vi "U8_3_byte_Array_to_voltage_current_Rev01.vi"(10 "Array In":u8[](array[numeric]), 11 "Nmbr_of_datasamples":dbl=128.0) -> (0 "Current":dbl[](graph), 1 "mV":dbl, 2 "Voltage":dbl[](graph), 3 "Loop count":dbl, 4 "COM":dbl[](graph), 6 "HEXVAL":string)   [LabVIEW 2012]
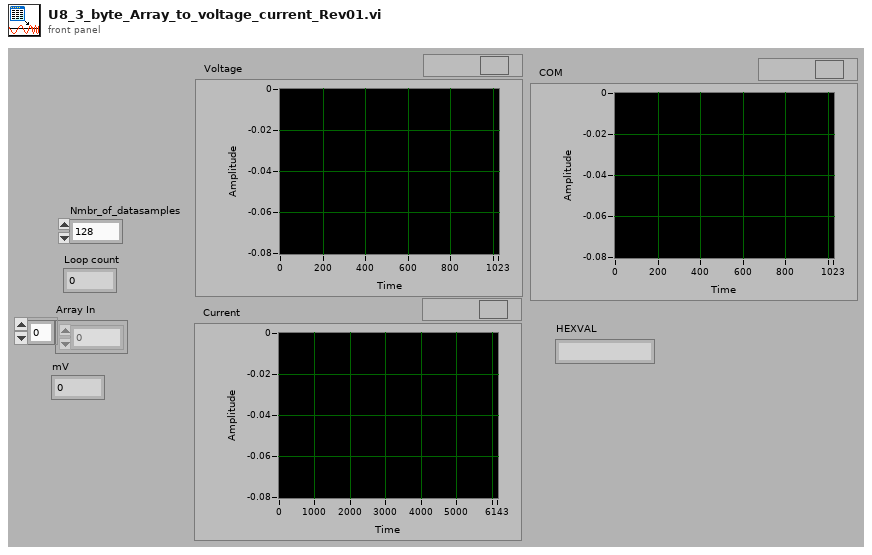
[diagram p1: front panel]
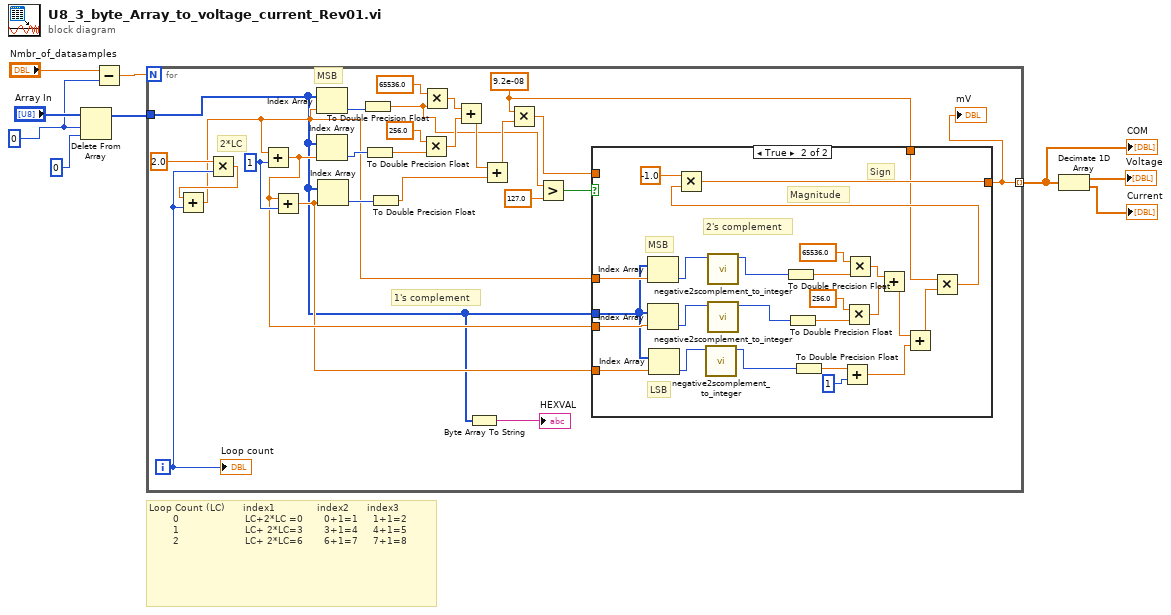
[diagram p0: block diagram]
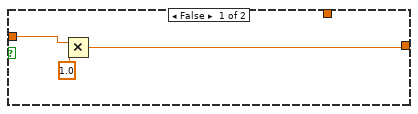
[diagram p2: hidden frame]
diagram:
  w5 = 0
  # "Loop Count (LC)      index1              index2      index3      \n        0                      LC+2*LC =0       0+1=1     1+1=2\n        1                      LC+ 2*LC=3       3+1=4     4+1=5\n        2                      LC+ 2*LC=6       6+1=7     7+1=8"
  n1 = Delete From Array(array="Array In", length=w5, index=0) -> (array with subset deleted=w4:u8[])  [unwired: 1 out]
  n2 = Subtract(x="Nmbr_of_datasamples", y=w5) -> (x-y=w7:dbl)
  n3 = for {
    N: w7 -> [_]
    tunnel: w4 -> [w10]
    tunnel: [w12] -> w1 mode=indexing
    i -> [w17]
    w16 = 9.2e-08
    w27 = 1
    # "1's complement"
    # "MSB"
    # "2*LC"
    n4 = Multiply(x=2.0, y=w17) -> (x*y=w25:dbl)
    n5 = Add(x=w25, y=w17) -> (x+y=w15:dbl)
    n6 = Add(x=w15, y=w27) -> (x+y=w14:dbl)
    n7 = Add(x=w14, y=w27) -> (x+y=w13:dbl)
    n8 = Index Array(array=w10, index=w15) -> (element=w20:u8)
    n9 = Index Array(array=w10, index=w14) -> (element=w19:u8)
    n10 = Index Array(array=w10, index=w13) -> (element=w18:u8)
    n11 = To Double Precision Float(number=w20) -> (double precision float=w21:dbl)
    n12 = To Double Precision Float(number=w19) -> (double precision float=w33:dbl)
    n13 = To Double Precision Float(number=w18) -> (double precision float=w29:dbl)
    n14 = Multiply(x=256.0, y=w33) -> (x*y=w31:dbl)
    n15 = Multiply(x=65536.0, y=w21) -> (x*y=w35:dbl)
    n16 = Add(x=w35, y=w31) -> (x+y=w30:dbl)
    n17 = Byte Array To String(unsigned byte array=w10) -> (string=→"HEXVAL":string)
    n18 = Add(x=w30, y=w29) -> (x+y=w28:dbl)
    n19 = Multiply(x=w16, y=w28) -> (x*y=w24:dbl)
    n20 = Greater?(x=w21, y=127.0) -> (0:w23:bool)
    n21 = case shown="True" w23 {
      tunnel: [w38 w63] -> w12
      tunnel: w24 -> [w37 _]
      tunnel: w10 -> [_ w48]
      tunnel: w15 -> [_ w53]
      tunnel: w14 -> [_ w52]
      tunnel: w13 -> [_ w51]
      tunnel: w16 -> [_ w49]
      frame False {
        n22 = Multiply(x=w37, y=1.0) -> (x*y=w38:dbl)
      }
      frame True {
        # "LSB"
        # "Magnitude"
        # "Sign"
        # "2's complement"
        # "MSB"
        n23 = Index Array(array=w48, index=w53) -> (element=w47:u8)
        n24 = Index Array(array=w48, index=w52) -> (element=w45:u8)
        n25 = Index Array(array=w48, index=w51) -> (element=w43:u8)
        n26 = call "negative2scomplement_to_integer.vi"("BYTE"=w43) -> ("Result"=w42:u8)  [unwired: 10 in]
        n27 = call "negative2scomplement_to_integer.vi"("BYTE"=w47) -> ("Result"=w46:u8)  [unwired: 10 in]
        n28 = call "negative2scomplement_to_integer.vi"("BYTE"=w45) -> ("Result"=w44:u8)  [unwired: 10 in]
        n29 = To Double Precision Float(number=w46) -> (double precision float=w54:dbl)
        n30 = To Double Precision Float(number=w44) -> (double precision float=w59:dbl)
        n31 = To Double Precision Float(number=w42) -> (double precision float=w41:dbl)
        n32 = Add(x=w41, y=1) -> (x+y=w40:dbl)
        n33 = Multiply(x=256.0, y=w59) -> (x*y=w57:dbl)
        n34 = Multiply(x=65536.0, y=w54) -> (x*y=w61:dbl)
        n35 = Add(x=w61, y=w57) -> (x+y=w56:dbl)
        n36 = Add(x=w56, y=w40) -> (x+y=w55:dbl)
        n37 = Multiply(x=w49, y=w55) -> (x*y=w50:dbl)
        n38 = Multiply(x=-1.0, y=w50) -> (x*y=w63:dbl)
      }
    }
    "mV" <- w12
    "Loop count" <- w17
  }
  "COM" <- w1
  n39 = Decimate 1D Array(w1) -> (→"Voltage":dbl[], →"Current":dbl[])
